vi "ramp for torque lr mode.vi"(9 "Current Sequence in":u16, 10 "ItemNames":string[][](array[string]), 11 "Torque":dbl) -> (2 "ramp":bool, 3 "Array":dbl[](array[numeric]))   [LabVIEW 2018]
uses:
  <vilib>/Analysis/1siggen.llb/Ramp Pattern by Delta.vi
  <vilib>/Analysis/NI_AALBase.lvlib
panel:
  out "Torque 2":dbl
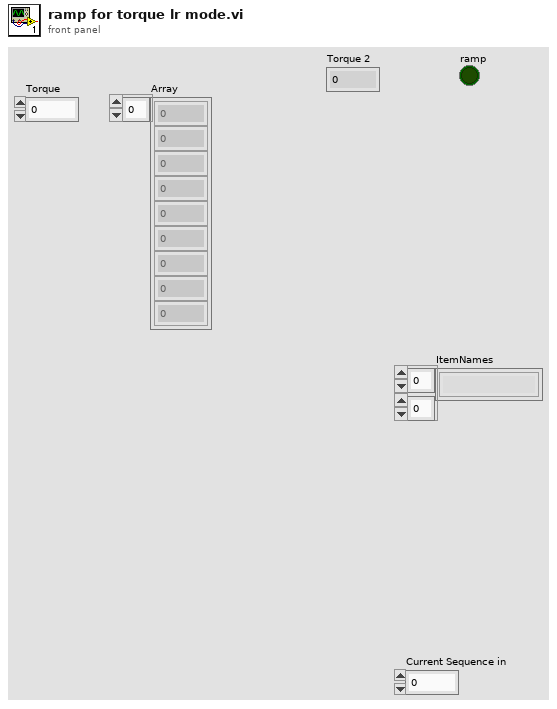
[diagram p1: front panel]
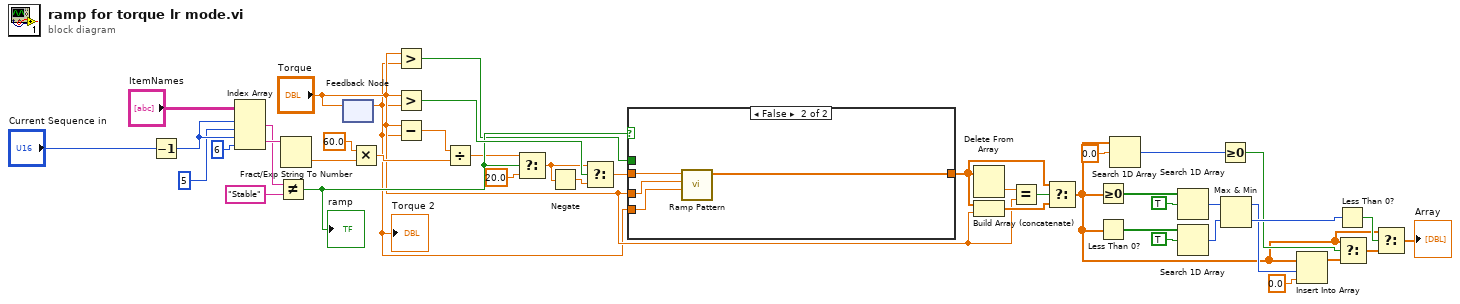
[diagram p0: block diagram]
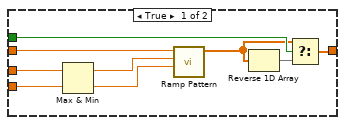
[diagram p2: hidden frame]
diagram:
  n1 = Decrement(x="Current Sequence in") -> (x-1=w16:u16)
  n2 = Index Array(array="ItemNames", index (row) #1=w16, index (col) #1=5 ("disabled index (col)"), index (row) #2=w16, index (col) #2=6 ("disabled index (col)")) -> (element #1=w12:string, element #2=w14:string)
  n3 = Not Equal?(x=w12, y="Stable") -> (x != y?=w7:bool)
  "ramp" <- w7
  n4 = Fract/Exp String To Number(string=w14) -> (number=w13:dbl)  [unwired: 3 in, 1 out]
  n5 = feedback-in #1("Torque") -> ()
  n6 = feedback #1() -> (w2:dbl)  [unwired: 1 in]
  "Torque 2" <- w2
  n7 = Multiply(x=60.0, y=w13) -> (x*y=w8:dbl)
  n8 = Greater?(x="Torque", y=w2) -> (0:w1:bool)
  n9 = Greater?(x="Torque", y=w2) -> (0:w43:bool)
  n10 = Subtract(x="Torque", y=w2) -> (x-y=w9:dbl)
  n11 = Divide(x=w9, y=w8) -> (x/y=w5:dbl)
  n12 = Select(t=w5, s=w7, f=20.0 ("t")) -> (s? t:f=w6:dbl)
  n13 = Negate(x=w6) -> (-x=w42:dbl)
  n14 = Select(t=w6, s=w43, f=w42) -> (s? t:f=w41:dbl)
  n15 = case shown="False" w7 {
    tunnel: w41 -> [w52 w56]
    tunnel: [w44 w55] -> w37
    tunnel: "Torque" -> [w51 w54]
    tunnel: w2 -> [w50 w53]
    tunnel: w1 -> [w47 _]
    frame True {
      n16 = Max & Min(x=w51, y=w50) -> (max(x,y)=w49:dbl, min(x,y)=w48:dbl)
      n17 = call-poly <vilib>:"Ramp Pattern.vi"("start"=w48, "end"=w49, "delta"=w52) -> ("Ramp Pattern"=w46:dbl[])  [unwired: 6 in, 2 out]
      n18 = Reverse 1D Array(array=w46) -> (reversed array=w45:dbl[])
      n19 = Select(t=w46, s=w47, f=w45) -> (s? t:f=w44:dbl[])
    }
    frame False {
      n20 = call-poly <vilib>:"Ramp Pattern.vi"("start"=w53, "end"=w54, "delta"=w56) -> ("Ramp Pattern"=w55:dbl[])  [unwired: 6 in, 2 out]
    }
  }
  n21 = Delete From Array(array=w37) -> (deleted portion=w40:dbl)  [unwired: 2 in, 1 out]
  n22 = Build Array (concatenate)(w37, "Torque") -> (w38:dbl[])
  n23 = Equal?(x=w40, y="Torque") -> (x = y?=w39:bool)
  n24 = Select(t=w37, s=w39, f=w38) -> (s? t:f=w22:dbl[])
  n25 = Greater Or Equal To 0?(x=w22) -> (x >= 0?=w36:bool[])
  n26 = Less Than 0?(x=w22) -> (x < 0?=w33:bool[])
  n27 = Search 1D Array(1D array=w22, element=0.0) -> (index of element=w24:i32)  [unwired: 1 in]
  n28 = Search 1D Array(1D array=w36, element=TRUE) -> (index of element=w32:i32)  [unwired: 1 in]
  n29 = Search 1D Array(1D array=w33, element=TRUE) -> (index of element=w31:i32)  [unwired: 1 in]
  n30 = Greater Or Equal To 0?(x=w24) -> (x >= 0?=w23:bool)
  n31 = Max & Min(x=w32, y=w31) -> (max(x,y)=w28:i32, min(x,y)=w30:i32)
  n32 = Insert Into Array(array=w22, index=w28, new element=0.0 ("new element/subarray")) -> (w21:dbl[])
  n33 = Less Than 0?(x=w30) -> (x < 0?=w29:bool)
  n34 = Select(t=w22, s=w23, f=w21) -> (s? t:f=w20:dbl[])
  n35 = Select(t=w22, s=w29, f=w20) -> (s? t:f=→"Array":dbl[])
